vi "Not Sure.vi"   [LabVIEW 2014]
uses:
  <vilib>/rvi/interface/nirviReadWriteControl/nirviReadWriteControl.xnode
  <vilib>/rvi/interface/Simulation/niFpgaSimulationCallBeginRW.vi
  <vilib>/rvi/errors/niLvFpgaAdjustHostInterfaceError.vi
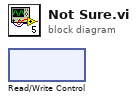
[diagram p0: block diagram]
diagram:
  n1 = xnode "Read/Write Control"() -> ("FPGA VI Reference In"=w1:refnum<k20>, "FPGA VI Reference Out"=w3:refnum<k20>, "error in"=w2:errorcluster, "error out"=w4:errorcluster)  [unwired: 1 out]
